vi "Compile HW Channel Data.vi"(8 "error in (no error)":errorcluster, 10 "Desired Values Refs":T1[](array[typedef]) format="%.0x", 11 "Device ref":T1 format="%.0x") -> (0 "error out":errorcluster, 3 "Device ref dup":T1 format="%.0x", 5 "Compiled HW Channels":T2[](array[typedef]))   [LabVIEW 2023, in "NI 272x Resistive Simulation Custom Device Configuration.lvlib"]
uses:
  NI 272x Resistive Simulation Custom Device Configuration.lvlib
  <vilib>/NI VeriStand/Custom Device API/Custom Device Item Ref.ctl
  Controls/Compiled HW Channel.ctl
  Controls/Channel Mode.ctl
  <instrlib>/ni272xReferenceVIs/ni272xReferenceVIs.llb/ni272x Callendar-Van Dusen RTD Parameters.ctl
  Globals/Names.vi
  <vilib>/NI VeriStand/Custom Device API/Get Item Property (U16).vi
  NI 272x Resistive Simulation Custom Device Shared.lvlib
  <vilib>/NI VeriStand/Custom Device API/Custom Device API.lvlib
  <vilib>/NI VeriStand/Custom Device Tools/Custom Device Utility Library/Custom Device Utility Library.lvlib
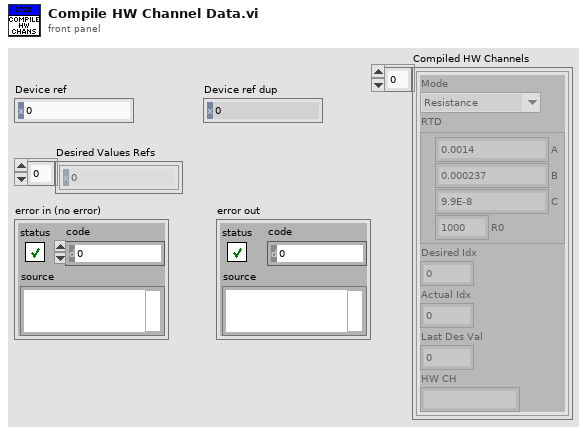
[diagram p1: front panel]
types:
  T1 = typedef "Custom Device API.lvlib/Custom Device Item Ref.ctl" = u64
  T2 = typedef "NI 272x Resistive Simulation Custom Device Shared.lvlib/Compiled HW Channel.ctl" = cluster{"Mode":T3, "RTD":T4, "Desired Idx":i32, "Actual Idx":i32, "Last Des Val":dbl, "HW CH":string}
  T3 = typedef "NI 272x Resistive Simulation Custom Device Shared.lvlib/Channel Mode.ctl" = enum16{"Resistance", "RTD Temperature"}
  T4 = typedef "ni272x Callendar-Van Dusen RTD Parameters.ctl" = cluster{"A":dbl, "B":dbl, "C":dbl, "R0":dbl}
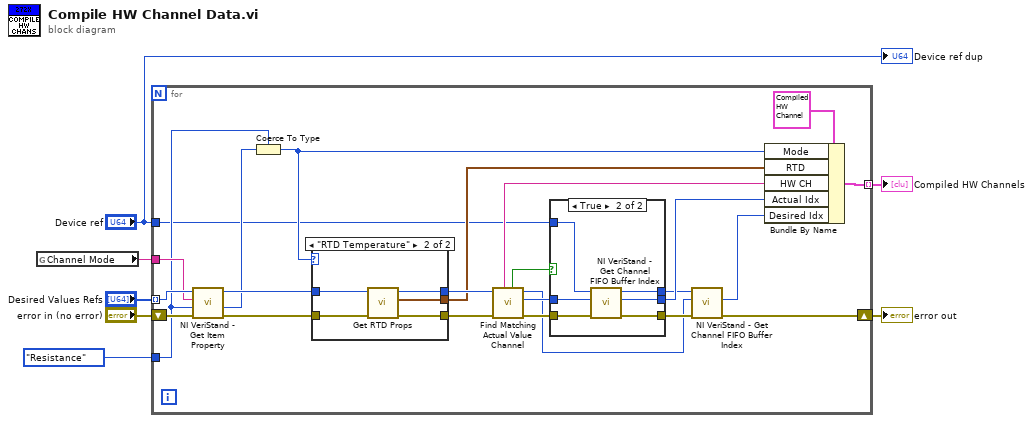
[diagram p0: block diagram]
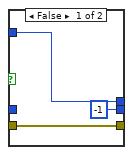
[diagram p2: hidden frame]
diagram:
  n1 = global read "Names.vi" "Channel Mode"() -> (w6:string)
  n2 = for {
    tunnel: "Desired Values Refs" -> [w28] mode=indexing
    tunnel: w6 -> [w27]
    tunnel: Channel_Mode."Resistance" ("Mode") -> [w22]
    tunnel: "Device ref" -> [w17]
    shift-right: [w10] -> w3
    shift-left: "error in (no error)" -> [w31]
    tunnel: [w9] -> w2 mode=indexing
    n3 = call-poly <vilib>:"NI VeriStand - Get Item Property.vi"("error in (no error)"=w31, "Default Value"=w22, "Property Name"=w27, "Item Ref in"=w28) -> ("error out"=w29:errorcluster, "Value"=w23:u16, "Item Ref out"=w25:T1)  [unwired: 4 in, 1 out]
    n4 = Coerce To Type(0:w23, 1:w22) -> (2:w21:T3)
    n5 = case shown="\"RTD Temperature\"" w21 {
      tunnel: w29 -> [w42 w47]
      tunnel: [w42 w46] -> w26
      tunnel: w25 -> [w41 w45]
      tunnel: [w41 w44] -> w24
      tunnel: [_ w43] -> w20
      frame "Resistance" {
      }
      frame "RTD Temperature" {
        n6 = call "Get RTD Props.vi"("error in (no error)"=w47, "Item Ref in"=w45) -> ("error out"=w46:errorcluster, "temp param"=w43:T4, "Item Ref out"=w44:T1)  [unwired: 7 in]
      }
    }
    n7 = call "Find Matching Actual Value Channel.vi"("error in (no error)"=w26, "Desired item ref in"=w24) -> ("error out"=w18:errorcluster, "Actual item ref"=w15:T1, "Desired item ref out"=w11:T1, "found"=w8:bool, "CH#"=w19:string)  [unwired: 4 in, 1 out]
    n8 = case shown="True" w8 {
      tunnel: w18 -> [w33 w40]
      tunnel: w15 -> [_ w38]
      tunnel: w17 -> [w32 w39]
      tunnel: [w33 w37] -> w14
      tunnel: [-1 ("Channel FIFO Buffer Index") w36] -> w16
      tunnel: [w32 w35] -> w13
      frame False {
      }
      frame True {
        n9 = call <vilib>:"NI VeriStand - Get Channel FIFO Buffer Index.vi"("error in"=w40, "Channel Ref"=w38, "Device Ref in"=w39) -> ("error out"=w37:errorcluster, "Channel FIFO Buffer Index"=w36:i32, "Device Ref out"=w35:T1)  [unwired: 4 in, 2 out]
      }
    }
    n10 = call <vilib>:"NI VeriStand - Get Channel FIFO Buffer Index.vi"("error in"=w14, "Channel Ref"=w11, "Device Ref in"=w13) -> ("error out"=w10:errorcluster, "Channel FIFO Buffer Index"=w12:i32)  [unwired: 4 in, 3 out]
    n11 = Bundle By Name(cluster=T2 {"Mode"=enum."Resistance", "RTD"={"A"=0.0, "B"=0.0, "C"=0.0, "R0"=0.0}, "Desired Idx"=0, "Actual Idx"=0, "Last Des Val"=0.0, "HW CH"=""} ("HW Chn"), "Mode"=w21, "RTD"=w20, "HW CH"=w19, "Actual Idx"=w16, "Desired Idx"=w12) -> (w9:T2)
  }
  "error out" <- w3
  "Compiled HW Channels" <- w2
  "Device ref dup" <- "Device ref"
